vi "getParameter.vi"(6 "DeviceParm":u8[](array[numeric]), 7 "Device handle":i32, 8 "error in (no error)":errorcluster, 9 "RequiredSizeInput":u32, 10 "Size":u32, 11 "SEDSpectrometer in":refnum<class "SEDSpectrometer.lvclass">) -> (0 "error out":errorcluster, 1 "DeviceParam":u8[](array[numeric]), 2 "RequiredSizeOutput":u32, 3 "SEDSpectrometer out":refnum<class "SEDSpectrometer.lvclass">, 5 "Output Value":i32)   [LabVIEW 2016, in "SEDSpectrometer.lvclass"]
uses:
  SEDSpectrometer.lvclass
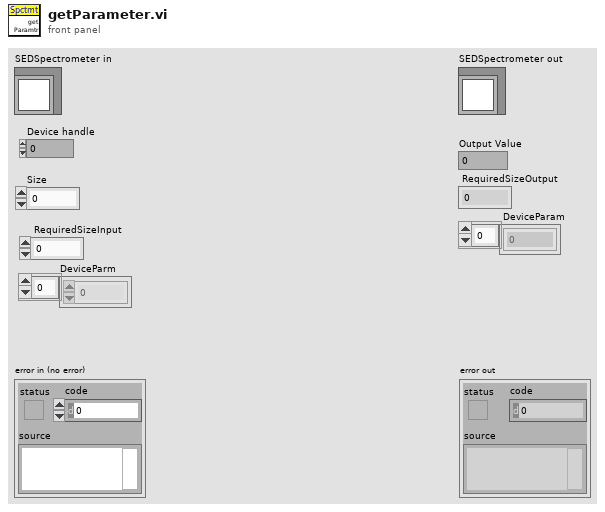
[diagram p1: front panel]
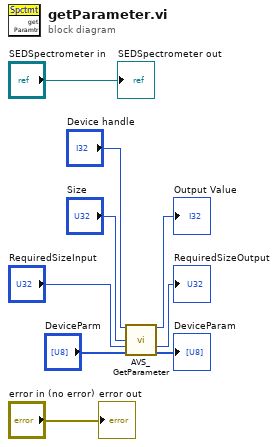
[diagram p0: block diagram]
diagram:
  n1 = call "AVS_GetParameter.vi"("a_hDevice"="Device handle", "a_Size"="Size", "RequiredSizeInput"="RequiredSizeInput", "DeviceParm"="DeviceParm") -> ("Output Value"=→"Output Value":i32, "RequiredSizeOutput"=→"RequiredSizeOutput":u32, "DeviceParam"=→"DeviceParam":u8[])  [unwired: 9 in]
  "error out" <- "error in (no error)"
  "SEDSpectrometer out" <- "SEDSpectrometer in"
